vi "Extract command and data from spreadsheet.vi"(8 "error in":errorcluster, 11 "Data spreadsheet":string[](array[string])) -> (0 "error out":errorcluster, 1 "Data":u32[](array[numeric]) format="%.0x", 2 "Command":u32 format="%.0x")   [LabVIEW 2019]
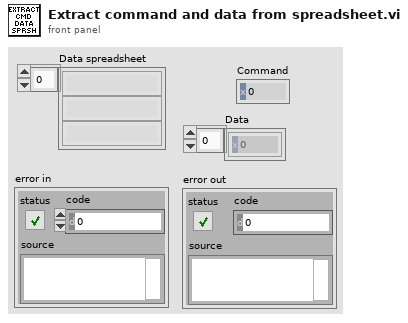
[diagram p1: front panel]
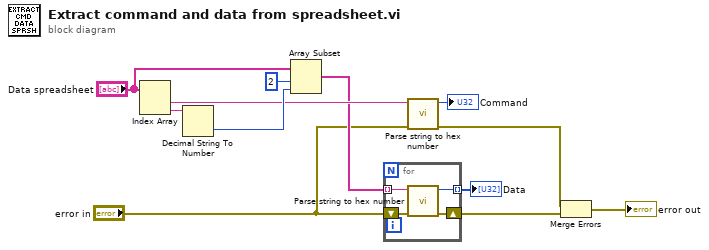
[diagram p0: block diagram]
diagram:
  n1 = Index Array(array="Data spreadsheet") -> (element #1=w8:string, element #2=w9:string)  [unwired: 2 in]
  n2 = Decimal String To Number(string=w9) -> (number=w12:i32)  [unwired: 2 in, 1 out]
  n3 = Array Subset(array="Data spreadsheet", index=2, length=w12) -> (w7:string[])
  n4 = for {
    tunnel: w7 -> [w16] mode=indexing
    tunnel: [w15] -> w1 mode=indexing
    shift-right: [w13] -> w6
    shift-left: "error in" -> [w14]
    n5 = call "Parse string to hex number.vi"("error in (no error)"=w14, "String"=w16) -> ("error out"=w13:errorcluster, "Numeric"=w15:u32)  [unwired: 8 in]
  }
  "Data" <- w1
  n6 = call "Parse string to hex number.vi"("error in (no error)"="error in", "String"=w8) -> ("error out"=w3:errorcluster, "Numeric"=→"Command":u32)  [unwired: 8 in]
  n7 = Merge Errors(w3, w6) -> (→"error out":errorcluster)
